vi "ITR LP.vi"(7 "input":dbl format="%.2f", 13 "corner period (steps)":dbl(slide)=10.237739663395852 scale=1.0..1000.0) -> (8 "output":dbl format="%.2f")   [LabVIEW 2017]
doc: "Modular ITR first order low pass filter with internal shift registers."
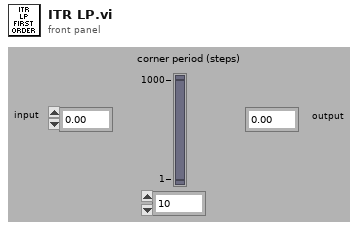
[diagram p1: front panel]
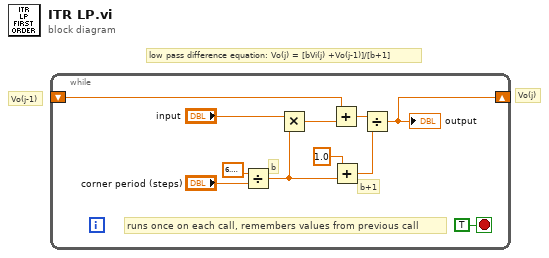
[diagram p0: block diagram]
diagram:
  # "Vo(j-1)"
  # "Vo(j)"
  # "low pass difference equation: Vo(j) = [bVi(j) +Vo(j-1)]/[b+1]"
  n1 = while {
    shift-left: _ -> [w1]
    shift-right: [w3] -> _
    stop <- TRUE stop-if-true
    # "b+1"
    # "b"
    # "runs once on each call, remembers values from previous call"
    n2 = Divide(x=6.283185307179586, y="corner period (steps)") -> (x/y=w6:dbl)
    n3 = Multiply(x="input", y=w6) -> (x*y=w2:dbl)
    n4 = Add(x=w1, y=w2) -> (x+y=w5:dbl)
    n5 = Add(x=1.0, y=w6) -> (x+y=w4:dbl)
    n6 = Divide(x=w5, y=w4) -> (x/y=w3:dbl)
    "output" <- w3
  }
